vi "writeParameterXML.vi"(8 "error in (no error)":errorcluster, 11 "ScriptEvent in":refnum<class "ScriptEvent.lvclass">) -> (0 "error out":errorcluster, 3 "ScriptEvent out":refnum<class "ScriptEvent.lvclass">)   [LabVIEW 2009, in "Tools.lvlib" / "Scripting.lvlib" / "ScriptEvent.lvclass"]
uses:
  ScriptEvent.lvclass
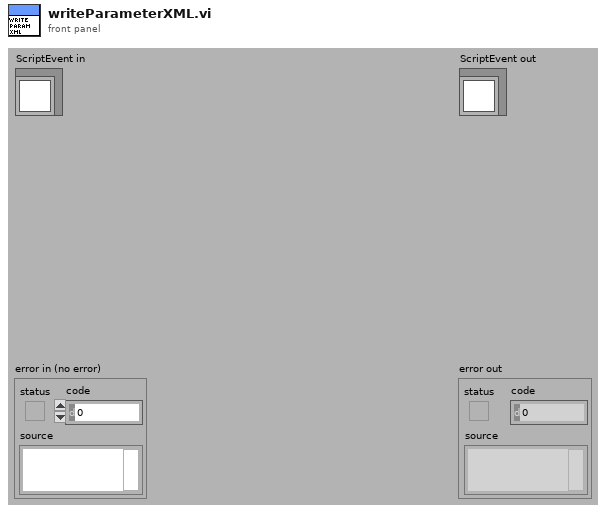
[diagram p1: front panel]
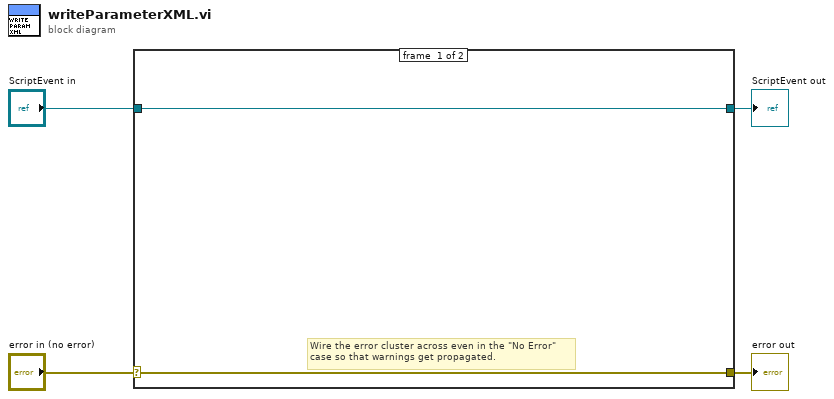
[diagram p0: block diagram]
diagram:
  n1 = case shown="No Error" "error in (no error)" {
    selector: "error in (no error)" -> [w5 w8]
    tunnel: [w5 w8] -> w3
    tunnel: [w6 w7] -> w1
    tunnel: "ScriptEvent in" -> [w6 w7]
    frame #0 {
      # "Wire the error cluster across even in the \"No Error\"\ncase so that warnings get propagated."
    }
    frame #1 {
    }
  }
  "error out" <- w3
  "ScriptEvent out" <- w1
